vi "Create Log11 emibin file.vi"(0 "file path":path, 5 "dbl Array":T1[](array[typedef]), 7 "u8 std Array":T2[](array[typedef]), 11 "error in":errorcluster, 12 "File type ID(0, generic)":u16, 13 "File type Version(0, Unset)":u8) -> (4 "refnum out":refnum<file>, 15 "error out":errorcluster)   [LabVIEW 2011]
uses:
  Ch Info u8 std.ctl
  Ch Info dbl.ctl
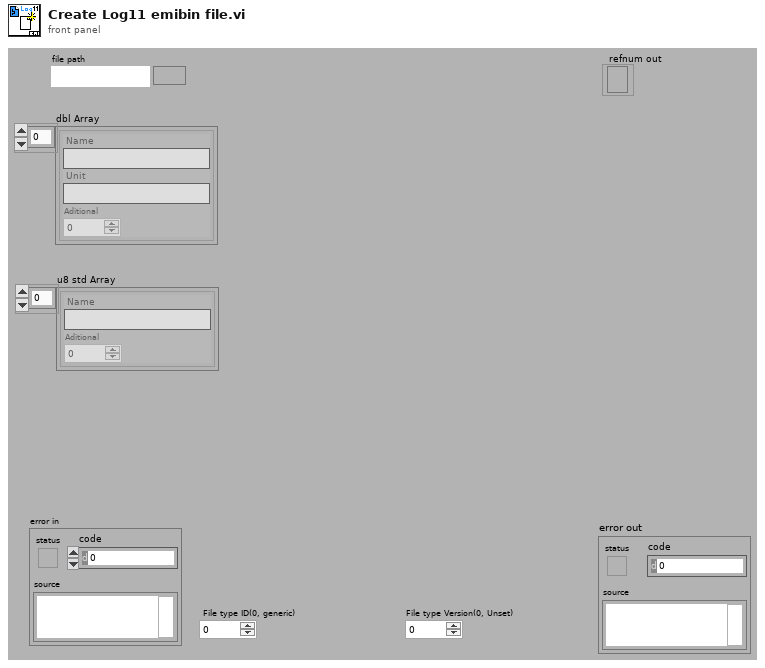
[diagram p1: front panel]
types:
  T1 = typedef "Ch Info dbl.ctl" = cluster{"Name":string, "Unit":string, "Aditional":i32}
  T2 = typedef "Ch Info u8 std.ctl" = cluster{"Name":string, "Aditional":i32}
  T3 = enum16{"big-endian, network order", "native, host order", "little-endian"}
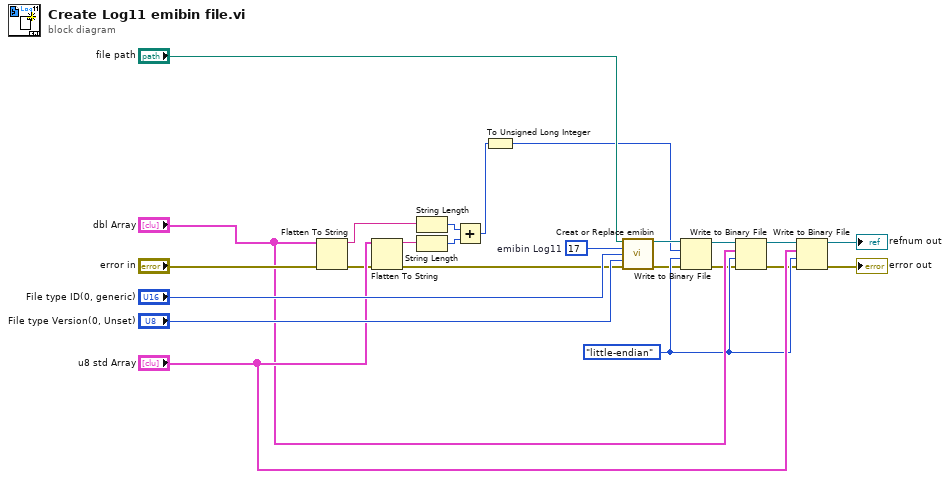
[diagram p0: block diagram]
diagram:
  w19 = T3."little-endian" ("byte order (0:big-endian, network order)")
  w6 = u8 17  # emibin Log11
  n1 = Flatten To String(anything="dbl Array", error in (no error)="error in") -> (data string=w4:string, error out=w1:errorcluster)  [unwired: 2 in, 1 out]
  n2 = Flatten To String(anything="u8 std Array", error in (no error)=w1) -> (data string=w5:string, error out=w7:errorcluster)  [unwired: 2 in, 1 out]
  n3 = String Length(string=w4) -> (length=w3:i32)
  n4 = String Length(string=w5) -> (length=w2:i32)
  n5 = Add(x=w3, y=w2) -> (x+y=w8:i32)
  n6 = To Unsigned Long Integer(number=w8) -> (unsigned 32bit integer=w10:u32)
  n7 = call "Creat or Replace emibin.vi"("file path"="file path", "File type Std(0)"=w6, "File type ID"="File type ID(0, generic)", "File type Version"="File type Version(0, Unset)", "error in (no error)"=w7) -> ("refnum out"=w11:refnum<file>, "error out"=w9:errorcluster)  [unwired: 9 in]
  n8 = Write to Binary File(file (use dialog)=w11, data=w10, error in=w9, 9:w19) -> (refnum out=w13:refnum<file>, error out=w12:errorcluster)  [unwired: 2 in, 1 out]
  n9 = Write to Binary File(file (use dialog)=w13, data="dbl Array", error in=w12, 9:w19) -> (refnum out=w15:refnum<file>, error out=w14:errorcluster)  [unwired: 2 in, 1 out]
  n10 = Write to Binary File(file (use dialog)=w15, data="u8 std Array", error in=w14, 9:w19) -> (refnum out=→"refnum out":refnum<file>, error out=→"error out":errorcluster)  [unwired: 2 in, 1 out]
